vi "显示UI.vi"() -> ()   [LabVIEW 2016, in "国弘多参数.lvlib"]
uses:
  <vilib>/Utility/miscctls.llb/LVPointTypeDef.ctl
  <vilib>/Utility/config.llb/NI_LVConfig.lvlib
panel:
  out "运行状态":u16(ring) items=["空闲", "水样测试", "标样核查"]
  in  "叶绿素a校准":bool
  in  "停止":bool
  in  "标样核查":bool
  in  "水样测试":bool
  in  "open MB":bool
  in  "设置":bool
  in  "水温校准":bool
  in  "浊度校准":bool
  in  "溶解氧校准":bool
  in  "电导率校准":bool
  in  "pH校准":bool
  in  "探头校正返回":bool
  in  "探头校正":bool
  in  "浊度参数查询":bool
  in  "溶解氧参数查询":bool
  in  "电导率参数查询":bool
  in  "pH参数查询":bool
  out "检测值":T1
  in  "返回":bool
  in  "参数查询":bool
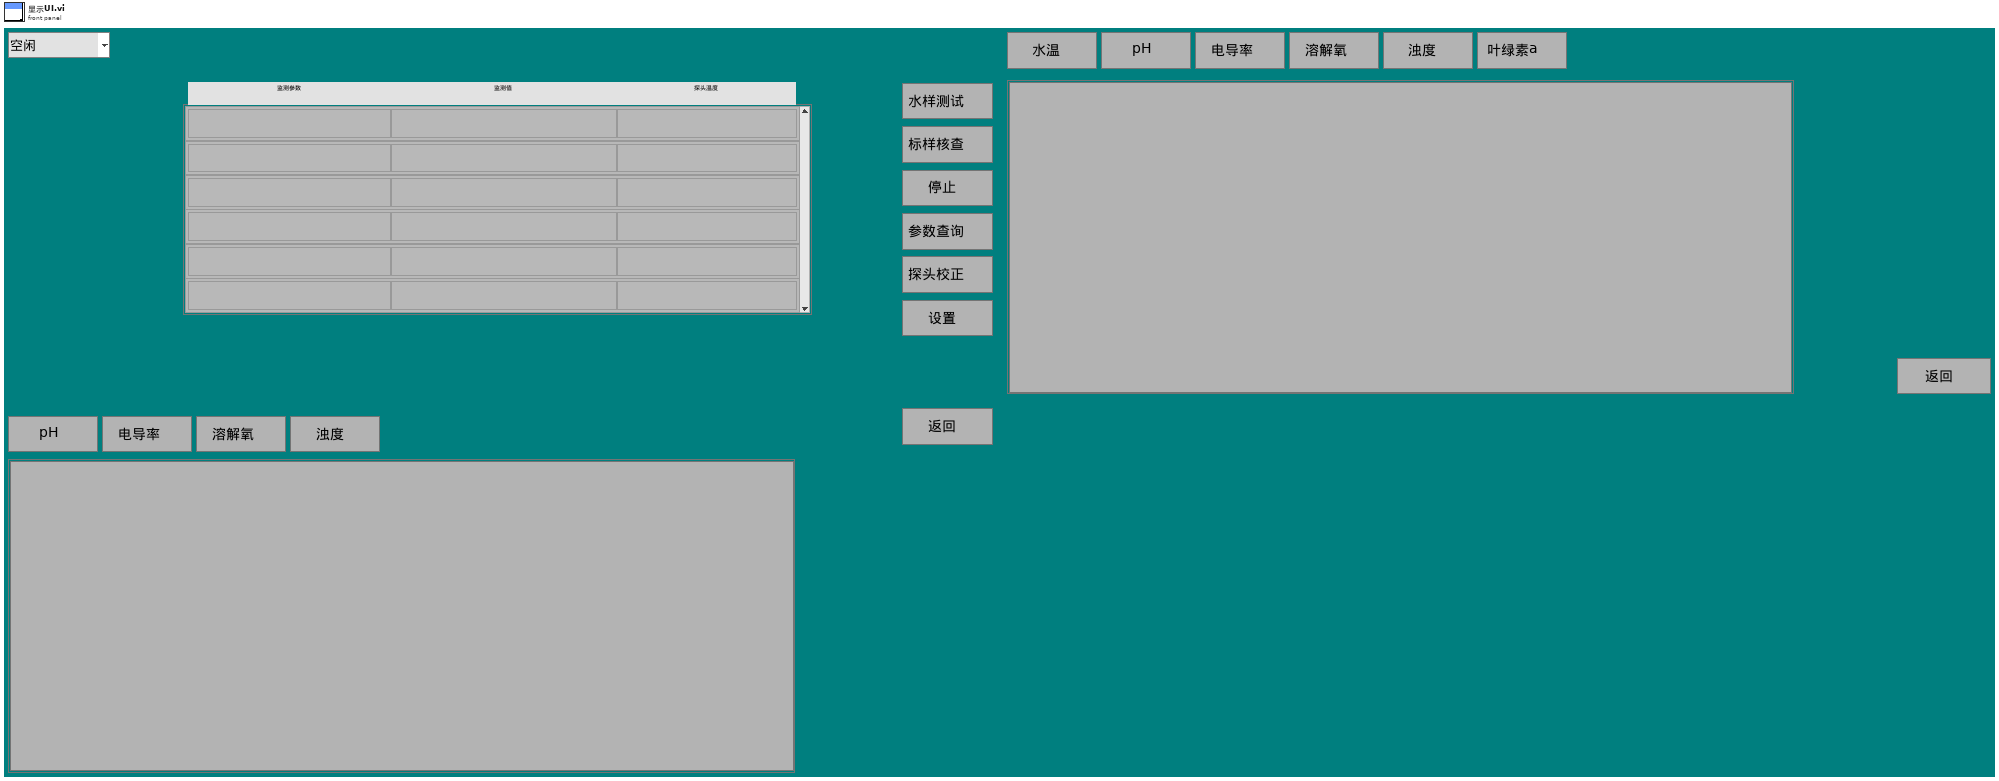
[diagram p1: front panel]
types:
  T1 = typedef "国弘多参数.lvlib/检测值.ctl" = cluster{"监测参数1":string, "浓度1":string, "探头温度1":string}[]
  T2 = typedef "LVPointTypeDef.ctl" = cluster{"Horizontal":i16, "Vertical":i16}
  T3 = cluster{"电极状态标志":u16, "电极型号标志":u16, "溶解氧测量值":sgl, "温度测量值":sgl, "溶解氧饱和度值":sgl, "盐度补偿值":sgl, "大气压补偿值":sgl, "溶解氧偏移修正值":sgl, "温度偏移修正值":sgl, "手动温度补偿值":sgl, "溶解氧电极零点":sgl, "溶解氧电极斜率":sgl, "第1点标准值记录":sgl, "第1点信号值记录":sgl, "第1点温度值记录":sgl, "第2点标准值记录":sgl, "第2点信号值记录":sgl, "第2点温度值记录":sgl, "命令滤波设定":u16, "温度模式":enum16{"ATC", "MTC"}, "生产批次":u16, "电极序号":u16, "串口地址":u16, "串口波特率":enum16{"9600", "19200", "115200"}, "串口校验位":enum16{"NONE", "ODD", "EVEN"}, "串口停止位":enum16{"1bit", "2bit"}, "第一点标准值":sgl, "第二点标准值":sgl}
  T4 = cluster{"电极状态标志":u16, "电极型号标志":u16, "酸碱度测量值":sgl, "温度测量值":sgl, "酸碱度信号值":sgl, "温度信号值":sgl, "酸碱度偏移修正值":sgl, "温度偏移修正值":sgl, "手动温度补偿值":sgl, "酸碱度电极零点":sgl, "酸碱度电极斜率":sgl, "第1点标准值记录":sgl, "第1点信号值记录":sgl, "第1点温度值记录":sgl, "第2点标准值记录":sgl, "第2点信号值记录":sgl, "第2点温度值记录":sgl, "命令滤波设定":u16, "温度模式":enum16{"ATC", "MTC"}, "生产批次":u16, "电极序号":u16, "串口地址":u16, "串口波特率":enum16{"9600", "19200", "115200"}, "串口校验位":enum16{"NONE", "ODD", "EVEN"}, "串口停止位":enum16{"1bit", "2bit"}, "第一点标准值":sgl, "第二点标准值":sgl}
  T5 = cluster{"电极状态标志":u16, "电极型号标志":u16, "浊度测量值":sgl, "温度测量值":sgl, "浊度信号值":sgl, "浊度偏移修正值":sgl, "温度偏移修正值":sgl, "手动温度补偿值":sgl, "浊度电极零点":sgl, "浊度电极斜率":sgl, "第1点标准值记录":sgl, "第1点信号值记录":sgl, "第1点温度值记录":sgl, "第2点标准值记录":sgl, "第2点信号值记录":sgl, "第2点温度值记录":sgl, "命令滤波设定":u16, "温度模式":enum16{"ATC", "MTC"}, "生产批次":u16, "电极序号":u16, "串口地址":u16, "串口波特率":enum16{"9600", "19200", "115200"}, "串口校验位":enum16{"NONE", "ODD", "EVEN"}, "串口停止位":enum16{"1bit", "2bit"}, "第一点标准值":sgl, "第二点标准值":sgl}
  T6 = cluster{"电极状态标志":u16, "电极型号标志":u16, "电导率测量值":sgl, "温度测量值":sgl, "电导率信号值":sgl, "温度信号值":sgl, "温度补偿系数":sgl, "电导率偏移修正值":sgl, "温度偏移修正值":sgl, "手动温度补偿值":sgl, "电导率电极零点":sgl, "电导率电极斜率":sgl, "命令滤波设定":u16, "温度模式":enum16{"ATC", "MTC"}, "生产批次":u16, "电极序号":u16, "串口地址":u16, "串口波特率":enum16{"9600", "19200", "115200"}, "串口校验位":enum16{"NONE", "ODD", "EVEN"}, "串口停止位":enum16{"1bit", "2bit"}, "第一点标准值":sgl, "第二点标准值":sgl}
  T7 = cluster{"监测参数1":string, "浓度1":string, "探头温度1":string}[]
  T8 = cluster{"CH":u16, "监测值":dbl, "监测信号值":dbl, "温度偏移修正值":sgl}
  T9 = typedef "NI_LVConfig.lvlib/Config Data RefNum.ctl" = refnum<k1>
  T10 = cluster{"baud rate (bps)":u32, "stop bits":u16, "parity":u16, "flow control":u16, "timeout":u32, "retries":i32}
  T11 = enum32{"Bad", "Idle", "Run top level", "Running"}
  T12 = cluster{"数据保存间隔":dbl, "水温标样值":dbl, "pH标样值":dbl, "溶解氧标样值":dbl, "电导率标样值":dbl, "浊度标样值":dbl}
  T13 = cluster{"Temp":bool, "pH":bool, "DO":bool, "Cond":bool, "Turb":bool, "叶绿素a启用":bool}
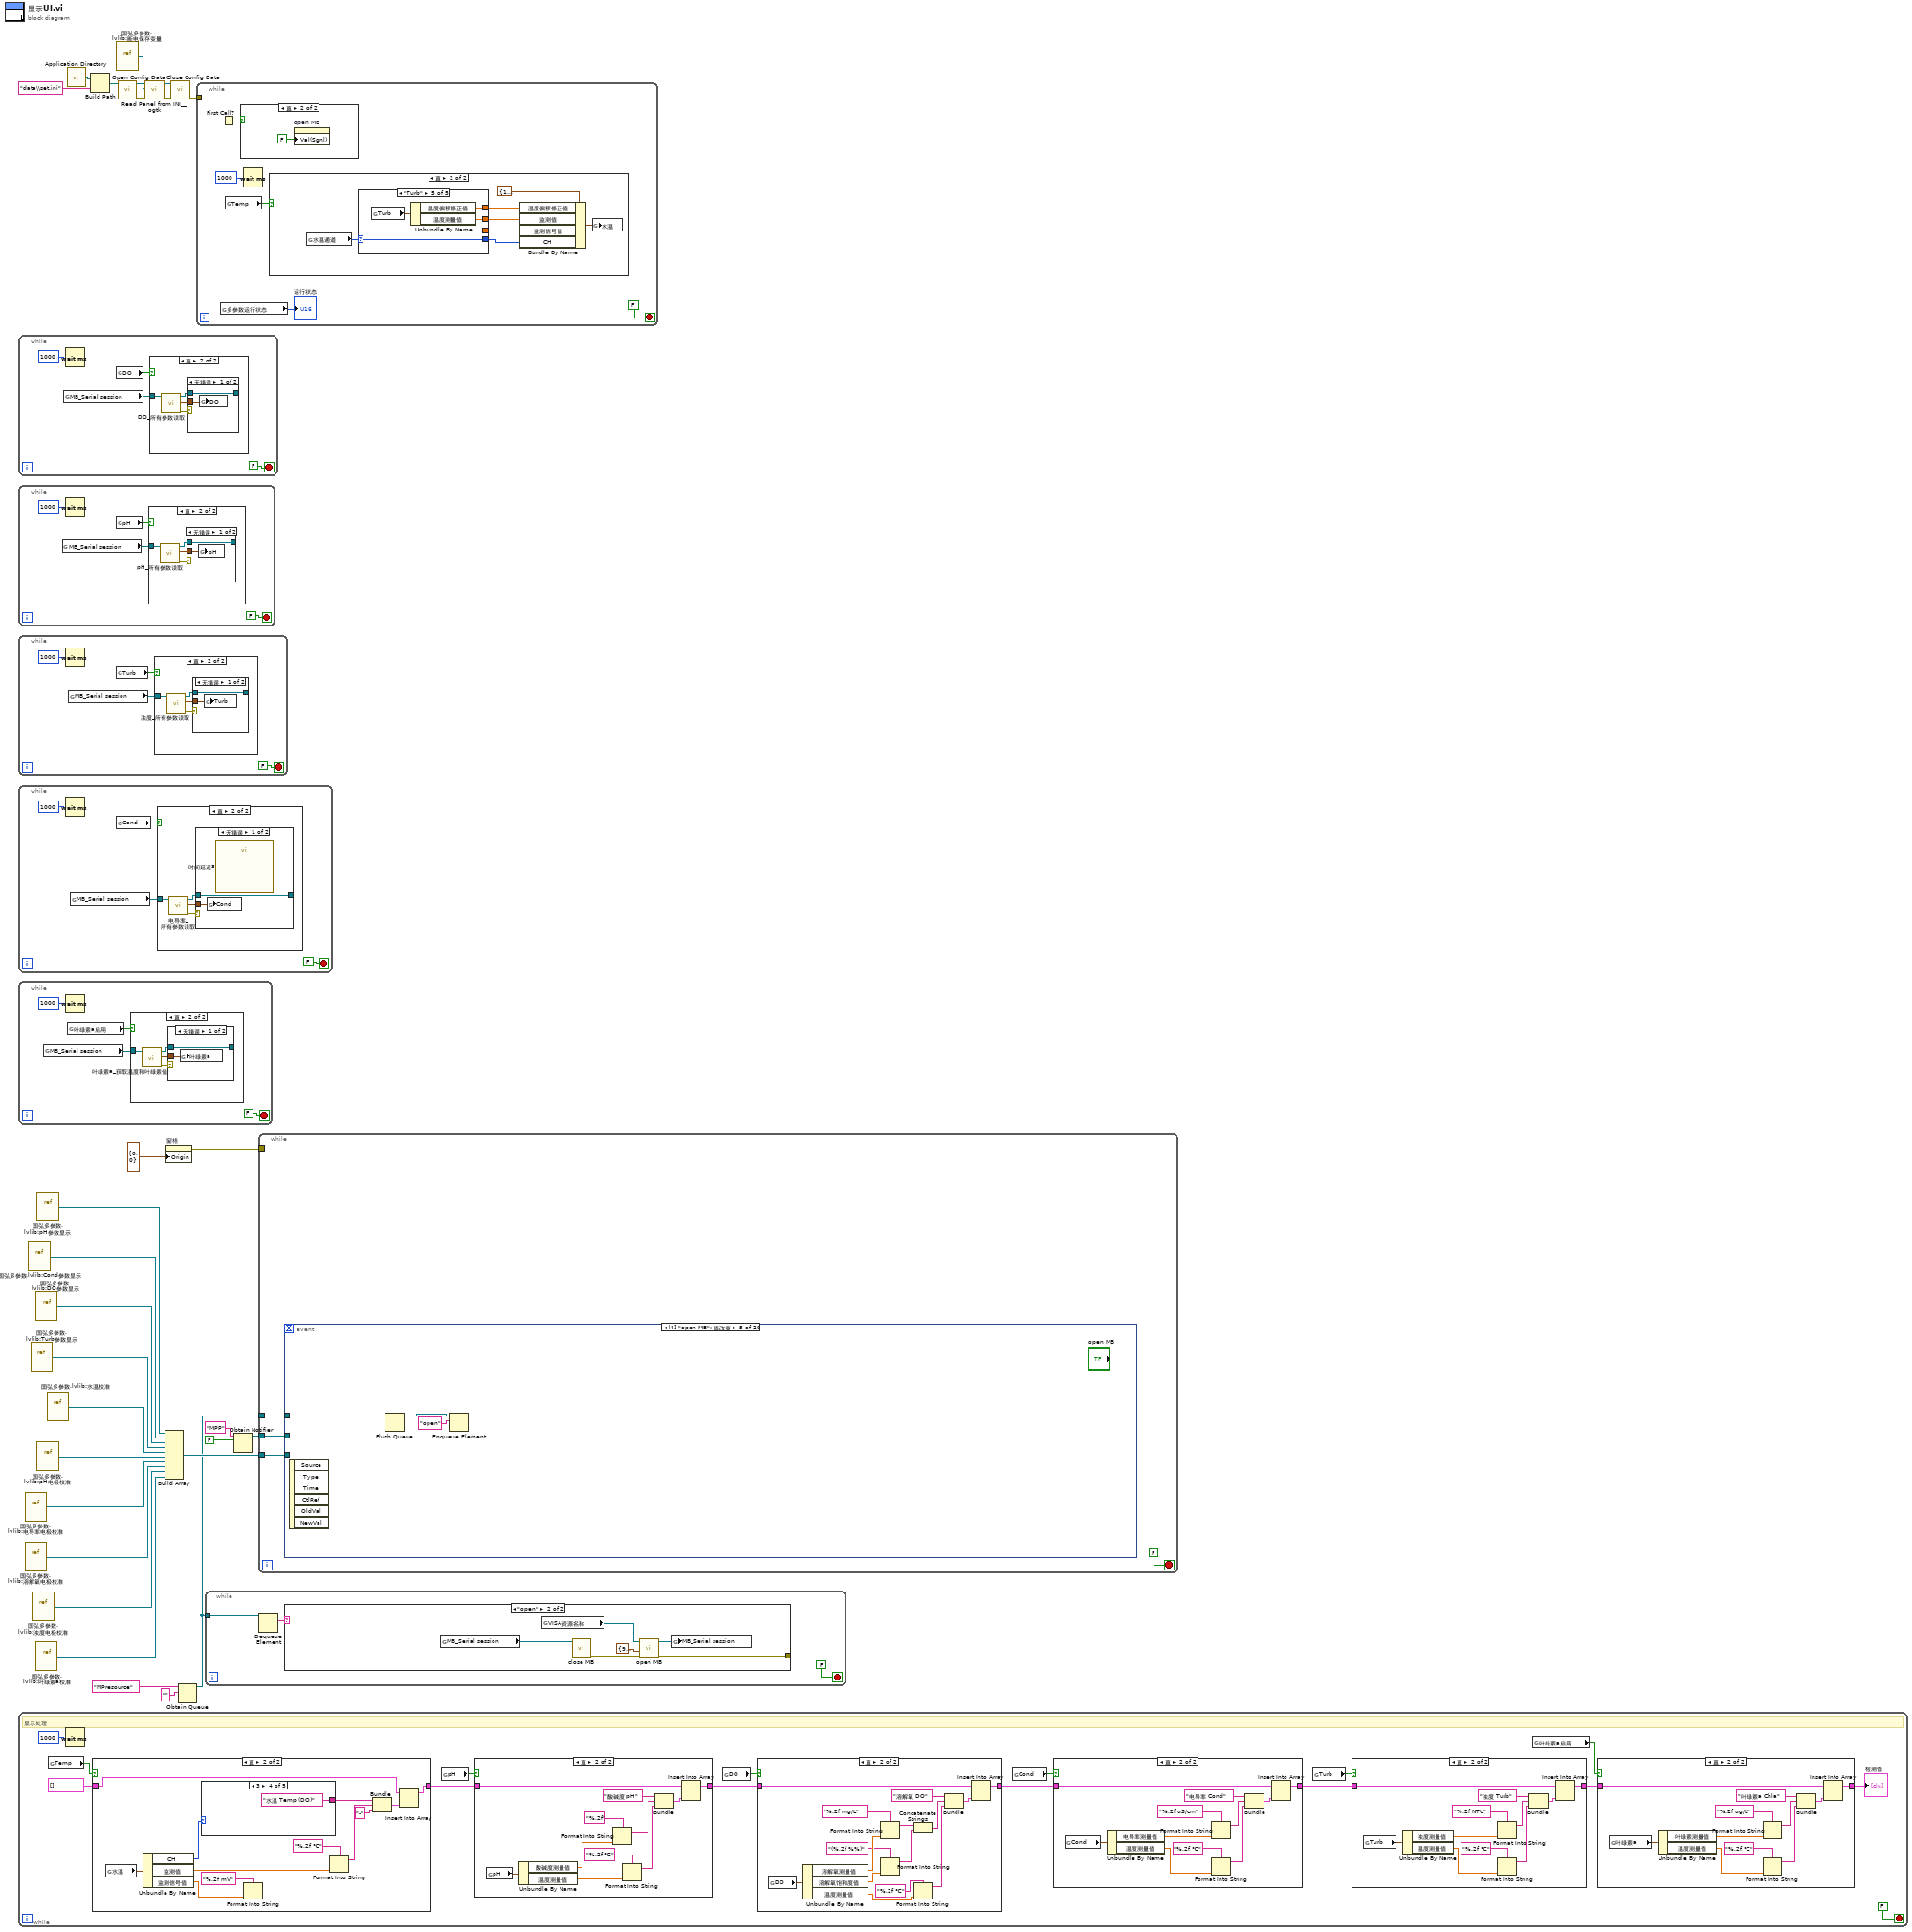
[diagram p0: block diagram]
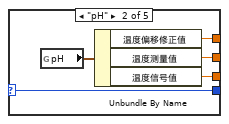
[diagram p15: hidden frame]
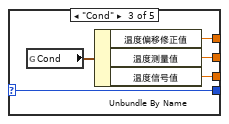
[diagram p16: hidden frame]
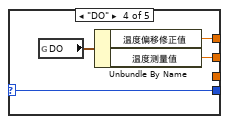
[diagram p17: hidden frame]
diagram:
  n1 = while {
    stop <- FALSE stop-if-true
    n2 = global read "过程全局变量.vi" "MB_Serial session"() -> (w29:refnum<class "MB_Master_Serial.lvclass">)
    n3 = Wait (ms)(milliseconds to wait=u32 1000 ("等待时间（毫秒）")) -> ()  [unwired: 1 out]
    n4 = global read "断电保存变量.vi" "DO"() -> (w30:bool)
    n5 = case shown="真" w30 {
      tunnel: w29 -> [_ w33]
      frame False {
      }
      frame True {
        n6 = call "DO_所有参数读取.vi"("MB_Serial session in"=w33) -> ("error out"=w35:errorcluster, "输出值"=w36:T3, "MB_Serial session out"=w34:refnum<class "MB_Master_Serial.lvclass">)  [unwired: 8 in]
        n7 = case shown="无错误" w35 {
          tunnel: w36 -> [w38 _]
          tunnel: w34 -> [w37 w39]
          tunnel: [w37 w39] -> _
          frame No Error {
            n8 = global write "过程全局变量.vi" "DO"(w38) -> ()
          }
          frame Error {
          }
        }
      }
    }
  }
  n9 = while {
    stop <- FALSE stop-if-true
    n10 = global read "过程全局变量.vi" "MB_Serial session"() -> (w41:refnum<class "MB_Master_Serial.lvclass">)
    n11 = Wait (ms)(milliseconds to wait=u32 1000 ("等待时间（毫秒）")) -> ()  [unwired: 1 out]
    n12 = global read "断电保存变量.vi" "pH"() -> (w42:bool)
    n13 = case shown="真" w42 {
      tunnel: w41 -> [_ w44]
      frame False {
      }
      frame True {
        n14 = call "pH_所有参数读取.vi"("MB_Serial session in"=w44) -> ("error out"=w46:errorcluster, "输出值"=w47:T4, "MB_Serial session out"=w45:refnum<class "MB_Master_Serial.lvclass">)  [unwired: 8 in]
        n15 = case shown="无错误" w46 {
          tunnel: w47 -> [w49 _]
          tunnel: w45 -> [w48 w50]
          tunnel: [w48 w50] -> _
          frame No Error {
            n16 = global write "过程全局变量.vi" "pH"(w49) -> ()
          }
          frame Error {
          }
        }
      }
    }
  }
  n17 = while {
    stop <- FALSE stop-if-true
    n18 = Wait (ms)(milliseconds to wait=u32 1000 ("等待时间（毫秒）")) -> ()  [unwired: 1 out]
    n19 = global read "过程全局变量.vi" "MB_Serial session"() -> (w52:refnum<class "MB_Master_Serial.lvclass">)
    n20 = global read "断电保存变量.vi" "Turb"() -> (w53:bool)
    n21 = case shown="真" w53 {
      tunnel: w52 -> [_ w55]
      frame False {
      }
      frame True {
        n22 = call "浊度_所有参数读取.vi"("MB_Serial session in"=w55) -> ("error out"=w57:errorcluster, "输出值"=w58:T5, "MB_Serial session out"=w56:refnum<class "MB_Master_Serial.lvclass">)  [unwired: 8 in]
        n23 = case shown="无错误" w57 {
          tunnel: w58 -> [w60 _]
          tunnel: w56 -> [w59 w61]
          tunnel: [w59 w61] -> _
          frame No Error {
            n24 = global write "过程全局变量.vi" "Turb"(w60) -> ()
          }
          frame Error {
          }
        }
      }
    }
  }
  n25 = while {
    stop <- FALSE stop-if-true
    n26 = Wait (ms)(milliseconds to wait=u32 1000 ("等待时间（毫秒）")) -> ()  [unwired: 1 out]
    n27 = global read "过程全局变量.vi" "MB_Serial session"() -> (w63:refnum<class "MB_Master_Serial.lvclass">)
    n28 = global read "断电保存变量.vi" "Cond"() -> (w64:bool)
    n29 = case shown="真" w64 {
      tunnel: w63 -> [_ w66]
      frame False {
      }
      frame True {
        n30 = call "电导率_所有参数读取.vi"("MB_Serial session in"=w66) -> ("error out"=w68:errorcluster, "输出值"=w69:T6, "MB_Serial session out"=w67:refnum<class "MB_Master_Serial.lvclass">)  [unwired: 8 in]
        n31 = case shown="无错误" w68 {
          tunnel: w69 -> [w71 _]
          tunnel: [w70 w72] -> _
          tunnel: w67 -> [w70 w72]
          frame No Error {
            n32 = global write "过程全局变量.vi" "Cond"(w71) -> ()
            n33 = call "时间延迟3"() -> ()  [unwired: 11 in, 1 out]
          }
          frame Error {
          }
        }
      }
    }
  }
  n34 = while {
    stop <- FALSE stop-if-true
    n35 = global read "过程全局变量.vi" "MB_Serial session"() -> (w75:refnum<class "MB_Master_Serial.lvclass">)
    n36 = Wait (ms)(milliseconds to wait=u32 1000 ("等待时间（毫秒）")) -> ()  [unwired: 1 out]
    n37 = global read "断电保存变量.vi" "叶绿素a启用"() -> (w74:bool)
    n38 = case shown="真" w74 {
      tunnel: w75 -> [_ w77]
      frame False {
      }
      frame True {
        n39 = call "叶绿素a_获取温度和叶绿素值.vi"("MB_Serial session in"=w77) -> ("error out"=w79:errorcluster, "输出值"=w80:cluster{"温度测量值":sgl, "叶绿素测量值":sgl, "错误标志":u16}, "MB_Serial session out"=w78:refnum<class "MB_Master_Serial.lvclass">)  [unwired: 8 in]
        n40 = case shown="无错误" w79 {
          tunnel: w80 -> [w82 _]
          tunnel: w78 -> [w81 w83]
          tunnel: [w81 w83] -> _
          frame No Error {
            n41 = global write "过程全局变量.vi" "叶绿素a"(w82) -> ()
          }
          frame Error {
          }
        }
      }
    }
  }
  n42 = while {
    stop <- FALSE stop-if-true
    # "显示处理"
    n43 = global read "断电保存变量.vi" "Temp"() -> (w96:bool)
    n44 = Wait (ms)(milliseconds to wait=u32 1000 ("等待时间（毫秒）")) -> ()  [unwired: 1 out]
    n45 = case shown="真" w96 {
      tunnel: [w163 w164] -> w93
      tunnel: T7 [] ("数组") -> [w163 w165]
      frame False {
      }
      frame True {
        n46 = global read "过程全局变量.vi" "水温"() -> (w175:T8)
        n47 = Unbundle By Name(w175) -> ("CH"=w170:u16, "监测值"=w173:dbl, "监测信号值"=w171:dbl)
        n48 = case shown="3" w170 {
          tunnel: ["水温 Temp" ("监测参数1") "水温 Temp (pH)" ("监测参数1") "水温 Temp (Cond)" ("监测参数1") "水温 Temp (DO)" ("监测参数1") "水温 Temp (Turb)" ("监测参数1")] -> w169
          frame 0, Default {
          }
          frame 1 {
          }
          frame 2 {
          }
          frame 3 {
          }
          frame 4 {
          }
        }
        n49 = Format Into String(format string="%.2f mV" ("格式字符串"), w171) -> ()  [unwired: 2 in, 2 out]
        n50 = Format Into String(format string="%.2f ℃" ("格式字符串"), w173) -> (resulting string=w168:string)  [unwired: 2 in, 1 out]
        n51 = Bundle("监测参数1"=w169, w168, "探头温度1"="-") -> (w166:cluster{"监测参数1":string, string, "探头温度1":string})  [unwired: 1 in]
        n52 = Insert Into Array(array=w165, new element=w166) -> (w164:T7)  [unwired: 1 in]
      }
    }
    n53 = global read "断电保存变量.vi" "pH"() -> (w94:bool)
    n54 = case shown="真" w94 {
      tunnel: [w151 w152] -> w91
      tunnel: w93 -> [w151 w154]
      frame False {
      }
      frame True {
        n55 = global read "过程全局变量.vi" "pH"() -> (w162:T4)
        n56 = Unbundle By Name(w162) -> ("酸碱度测量值"=w161:sgl, "温度测量值"=w159:sgl)
        n57 = Format Into String(format string="%.2f" ("格式字符串"), w161) -> (resulting string=w155:string)  [unwired: 2 in, 1 out]
        n58 = Format Into String(format string="%.2f ℃" ("格式字符串"), w159) -> (resulting string=w157:string)  [unwired: 2 in, 1 out]
        n59 = Bundle("监测参数2"="酸碱度 pH", w155, w157) -> (w153:cluster{"监测参数2":string, string, string})  [unwired: 1 in]
        n60 = Insert Into Array(array=w154, new element=w153) -> (w152:T7)  [unwired: 1 in]
      }
    }
    n61 = global read "断电保存变量.vi" "DO"() -> (w92:bool)
    n62 = case shown="真" w92 {
      tunnel: [w135 w136] -> w88
      tunnel: w91 -> [w135 w137]
      frame False {
      }
      frame True {
        n63 = global read "过程全局变量.vi" "DO"() -> (w146:T3)
        n64 = Unbundle By Name(w146) -> ("溶解氧测量值"=w147:sgl, "溶解氧饱和度值"=w144:sgl, "温度测量值"=w149:sgl)
        n65 = Format Into String(format string="%.2f mg/L" ("格式字符串"), w147) -> (resulting string=w143:string)  [unwired: 2 in, 1 out]
        n66 = Format Into String(format string="(%.2f %%)" ("格式字符串"), w144) -> (resulting string=w142:string)  [unwired: 2 in, 1 out]
        n67 = Concatenate Strings(w143, w142) -> (w141:string)
        n68 = Format Into String(format string="%.2f ℃" ("格式字符串"), w149) -> (resulting string=w139:string)  [unwired: 2 in, 1 out]
        n69 = Bundle("监测参数2"="溶解氧 DO", w141, w139) -> (w138:cluster{"监测参数2":string, string, string})  [unwired: 1 in]
        n70 = Insert Into Array(array=w137, new element=w138) -> (w136:T7)  [unwired: 1 in]
      }
    }
    n71 = global read "断电保存变量.vi" "Cond"() -> (w90:bool)
    n72 = case shown="真" w90 {
      tunnel: w88 -> [w123 w126]
      tunnel: [w123 w124] -> w87
      frame False {
      }
      frame True {
        n73 = global read "过程全局变量.vi" "Cond"() -> (w134:T6)
        n74 = Unbundle By Name(w134) -> ("电导率测量值"=w133:sgl, "温度测量值"=w131:sgl)
        n75 = Format Into String(format string="%.2f uS/cm" ("格式字符串"), w133) -> (resulting string=w127:string)  [unwired: 2 in, 1 out]
        n76 = Format Into String(format string="%.2f ℃" ("格式字符串"), w131) -> (resulting string=w128:string)  [unwired: 2 in, 1 out]
        n77 = Bundle("监测参数2"="电导率 Cond", w127, w128) -> (w125:cluster{"监测参数2":string, string, string})  [unwired: 1 in]
        n78 = Insert Into Array(array=w126, new element=w125) -> (w124:T7)  [unwired: 1 in]
      }
    }
    n79 = global read "断电保存变量.vi" "Turb"() -> (w89:bool)
    n80 = case shown="真" w89 {
      tunnel: w87 -> [w111 w114]
      tunnel: [w111 w112] -> w86
      frame False {
      }
      frame True {
        n81 = global read "过程全局变量.vi" "Turb"() -> (w118:T5)
        n82 = Unbundle By Name(w118) -> ("浊度测量值"=w119:sgl, "温度测量值"=w121:sgl)
        n83 = Format Into String(format string="%.2f NTU" ("格式字符串"), w119) -> (resulting string=w116:string)  [unwired: 2 in, 1 out]
        n84 = Format Into String(format string="%.2f ℃" ("格式字符串"), w121) -> (resulting string=w117:string)  [unwired: 2 in, 1 out]
        n85 = Bundle("监测参数2"="浊度 Turb", w116, w117) -> (w113:cluster{"监测参数2":string, string, string})  [unwired: 1 in]
        n86 = Insert Into Array(array=w114, new element=w113) -> (w112:T7)  [unwired: 1 in]
      }
    }
    n87 = global read "断电保存变量.vi" "叶绿素a启用"() -> (w84:bool)
    n88 = case shown="真" w84 {
      tunnel: w86 -> [w99 w102]
      tunnel: [w99 w100] -> w85
      frame False {
      }
      frame True {
        n89 = global read "过程全局变量.vi" "叶绿素a"() -> (w106:cluster{"温度测量值":sgl, "叶绿素测量值":sgl, "错误标志":u16})
        n90 = Unbundle By Name(w106) -> ("叶绿素测量值"=w107:sgl, "温度测量值"=w109:sgl)
        n91 = Format Into String(format string="%.2f ug/L" ("格式字符串"), w107) -> (resulting string=w104:string)  [unwired: 2 in, 1 out]
        n92 = Format Into String(format string="%.2f ℃" ("格式字符串"), w109) -> (resulting string=w105:string)  [unwired: 2 in, 1 out]
        n93 = Bundle("监测参数2"="叶绿素a Chla", w104, w105) -> (w101:cluster{"监测参数2":string, string, string})  [unwired: 1 in]
        n94 = Insert Into Array(array=w102, new element=w101) -> (w100:T7)  [unwired: 1 in]
      }
    }
    "检测值" <- w85
  }
  n95 = vi-ref "国弘多参数.lvlib:电导率电极校准.vi"() -> (w19:refnum<vi>)
  n96 = vi-ref "国弘多参数.lvlib:溶解氧电极校准.vi"() -> (w18:refnum<vi>)
  n97 = vi-ref "国弘多参数.lvlib:Cond参数显示.vi"() -> (w25:refnum<vi>)
  n98 = vi-ref "国弘多参数.lvlib:Turb参数显示.vi"() -> (w23:refnum<vi>)
  n99 = vi-ref "国弘多参数.lvlib:浊度电极校准.vi"() -> (w17:refnum<vi>)
  n100 = vi-ref "国弘多参数.lvlib:DO参数显示.vi"() -> (w24:refnum<vi>)
  n101 = vi-ref "国弘多参数.lvlib:叶绿素a校准.vi"() -> (w7:refnum<vi>)
  n102 = vi-ref "国弘多参数.lvlib:pH参数显示.vi"() -> (w26:refnum<vi>)
  n103 = vi-ref "国弘多参数.lvlib:pH电极校准.vi"() -> (w20:refnum<vi>)
  n104 = vi-ref "国弘多参数.lvlib:水温校准.vi"() -> (w21:refnum<vi>)
  n105 = call <vilib>:"Application Directory.vi"() -> ("Application Directory"=w12:path)
  n106 = Build Path(base path=w12, name or relative path="data\\set.ini" ("名称或相对路径")) -> (appended path=w11:path)
  n107 = vi-ref "国弘多参数.lvlib:断电保存变量.vi"() -> (w9:refnum<vi>)
  n108 = call <vilib>:"Open Config Data.vi"("configuration file path"=w11) -> ("error out"=w15:errorcluster, "refnum"=w16:T9)  [unwired: 8 in, 1 out]
  n109 = call <userlib>:"Read Panel from INI__ogtk.vi"("error in (no error)"=w15, "VI ref"=w9, "refnum"=w16) -> ("error out"=w13:errorcluster, "refnum out"=w14:T9)  [unwired: 7 in]
  n110 = Build Array(w26, w25, w24, w23, w21, w20, w19, w18, w17, w7) -> (w22:refnum<vi>[])
  n111 = property on="窗格" class="Pane"("Origin"=T2 {"Horizontal"=0, "Vertical"=0} ("原点")) -> (error out=w28:errorcluster)  [unwired: 2 in, 1 out]
  n112 = call <vilib>:"Close Config Data.vi"("error in (no error)"=w13, "refnum"=w14) -> ("error out"=w8:errorcluster)  [unwired: 8 in, 1 out]
  n113 = Obtain Queue(name (unnamed)="MPresource" ("名称（未命名）"), element data type="" ("名称（未命名）")) -> (queue out=w1:refnum<queue>)  [unwired: 3 in, 2 out]
  n114 = while {
    tunnel: w8 -> [_]
    stop <- FALSE stop-if-true
    n115 = First Call?() -> (First Call?: T/F=w183:bool)
    n116 = global read "过程全局变量.vi" "多参数运行状态"() -> (→"运行状态":u16)
    n117 = global read "断电保存变量.vi" "Temp"() -> (w182:bool)
    n118 = case shown="真" w183 {
      frame False {
      }
      frame True {
        n119 = property on="open MB" class="Bool (严格)"("Val(Sgnl)"=FALSE ("值(信号)")) -> ()  [unwired: 2 in, 2 out]
      }
    }
    n120 = Wait (ms)(milliseconds to wait=u32 1000 ("等待时间（毫秒）")) -> ()  [unwired: 1 out]
    n121 = case shown="真" w182 {
      frame False {
      }
      frame True {
        n122 = global read "断电保存变量.vi" "水温通道"() -> (w192:enum16{"NULL", "pH", "Cond", "DO", "Turb"})
        n123 = case shown="\"Turb\"" w192 {
          selector: w192 -> [w193 w198 w203 w207 w211]
          tunnel: [w193 w198 w203 w207 w211] -> w191
          tunnel: [_ w196 w201 w205 w209] -> w190
          tunnel: [_ w195 w200 _ _] -> w189
          tunnel: [_ w194 w199 w204 w208] -> w186
          frame "NULL", Default {
          }
          frame "pH" {
            n124 = global read "过程全局变量.vi" "pH"() -> (w197:T4)
            n125 = Unbundle By Name(w197) -> ("温度偏移修正值"=w194:sgl, "温度测量值"=w196:sgl, "温度信号值"=w195:sgl)
          }
          frame "Cond" {
            n126 = global read "过程全局变量.vi" "Cond"() -> (w202:T6)
            n127 = Unbundle By Name(w202) -> ("温度偏移修正值"=w199:sgl, "温度测量值"=w201:sgl, "温度信号值"=w200:sgl)
          }
          frame "DO" {
            n128 = global read "过程全局变量.vi" "DO"() -> (w206:T3)
            n129 = Unbundle By Name(w206) -> ("温度偏移修正值"=w204:sgl, "温度测量值"=w205:sgl)
          }
          frame "Turb" {
            n130 = global read "过程全局变量.vi" "Turb"() -> (w210:T5)
            n131 = Unbundle By Name(w210) -> ("温度偏移修正值"=w208:sgl, "温度测量值"=w209:sgl)
          }
        }
        n132 = Bundle By Name(cluster=T8 {"CH"=1, "监测值"=0.0, "监测信号值"=0.0, "温度偏移修正值"=0.0} ("水温"), "温度偏移修正值"=w186, "监测值"=w190, "监测信号值"=w189, "CH"=w191) -> (w188:T8)
        n133 = global write "过程全局变量.vi" "水温"(w188) -> ()
      }
    }
  }
  n134 = while {
    tunnel: w1 -> [w214]
    stop <- FALSE stop-if-true
    n135 = Dequeue Element(queue=w214) -> (element=w213:string)  [unwired: 2 in, 3 out]
    n136 = case shown="\"open\"" w213 {
      tunnel: [_ w216] -> _
      frame "假", Default {
      }
      frame "open" {
        n137 = global read "过程全局变量.vi" "MB_Serial session"() -> (w221:refnum<class "MB_Master_Serial.lvclass">)
        n138 = global read "断电保存变量.vi" "VISA资源名称"() -> (w218:refnum<visa-resource-name>)
        n139 = call "close MB.vi"("MB_Serial session"=w221) -> ("error out"=w220:errorcluster)  [unwired: 10 in]
        n140 = call "open MB.vi"("error in (no error)"=w220, "Serial Config"=T10 {"baud rate (bps)"=9600, "stop bits"=10, "parity"=0, "flow control"=0, "timeout"=1000, "retries"=1}, "VISA资源名称"=w218) -> ("error out"=w216:errorcluster, "MB_Serial session"=w219:refnum<class "MB_Master_Serial.lvclass">)  [unwired: 7 in]
        n141 = global write "过程全局变量.vi" "MB_Serial session"(w219) -> ()
      }
    }
  }
  n142 = Obtain Notifier(name (unnamed)="MPP" ("名称（未命名）"), notification data type=FALSE) -> (notifier out=w4:refnum<notifier>)  [unwired: 2 in, 2 out]
  n143 = while {
    tunnel: w28 -> [_]
    tunnel: w22 -> [w224]
    tunnel: w4 -> [w223]
    tunnel: w1 -> [w222]
    stop <- FALSE stop-if-true
    n144 = event shown="[4] \"open MB\": 值改变" {
      selector: _ -> [_ _ _ _ _ _ _ _ _ _ _ _ _ _ _ _ _ _ _ _]
      dyn-events: _ -> [_ _ _ _ _ _ _ _ _ _ _ _ _ _ _ _ _ _ _ _]
      timeout: _ -> [_ _ _ _ _ _ _ _ _ _ _ _ _ _ _ _ _ _ _ _]
      tunnel: w224 -> [_ _ _ _ _ _ w284 w297 w309 w317 w329 w341 w353 w365 w377 w389 w401 w413 w425 w437]
      tunnel: w223 -> [_ _ _ w257 _ _ _ _ _ _ _ _ _ _ _ _ _ _ _ _]
      tunnel: w222 -> [_ _ _ _ w260 _ _ _ _ _ _ _ _ _ _ _ _ _ _ _]
      event Timeout {
        n145 = event-data() -> ()  [unwired: 1 in, 3 out]
      }
      event "水样测试": Value Change {
        n146 = event-data() -> ()  [unwired: 1 in, 6 out]
        n147 = call "水样测试配置.vi"() -> ("确认输出"=w227:bool, "水样测定时间输出"=w226:dbl)  [unwired: 10 in]
        n148 = case shown="真" w227 {
          tunnel: w226 -> [_ w230]
          frame False {
          }
          frame True {
            n149 = vi-ref "国弘多参数.lvlib:水样测试.vi"() -> (w231:refnum<vi>)
            n150 = property class="VI"(reference=w231) -> ("Name"=w235:string, "Exec.State"=w233:T11)  [unwired: 1 in, 2 out]
            n151 = Open VI Reference(type specifier VI Refnum (for type only)=refnum<vi> refnum, vi path=w235, options=128 ("选项")) -> (vi reference=w236:refnum<vi>)  [unwired: 3 in, 1 out]
            n152 = case shown="\"Idle\"" w233 {
              tunnel: [w237 w241] -> w232
              tunnel: w236 -> [w237 w240]
              tunnel: w230 -> [_ w239]
              tunnel: "hd" ("数据标记表") -> [_ w238]
              frame "Bad", Default {
              }
              frame "Idle" {
                n153 = call-by-ref "开始异步调用"(reference=w240, "数据标记表"=w238, "水样测试时间"=w239) -> (reference out=w241:refnum<vi>)  [unwired: 11 in, 1 out]
              }
            }
            n154 = Close Reference(reference=w232) -> ()  [unwired: 1 in, 1 out]
          }
        }
      }
      event "标样核查": Value Change {
        n155 = event-data() -> ()  [unwired: 1 in, 6 out]
        n156 = call "标样核查配置.vi"() -> ("确认输出"=w243:bool, "标样核查配置"=w242:T12)  [unwired: 10 in]
        n157 = case shown="真" w243 {
          tunnel: w242 -> [_ w244]
          frame False {
          }
          frame True {
            n158 = vi-ref "国弘多参数.lvlib:标样核查.vi"() -> (w245:refnum<vi>)
            n159 = property class="VI"(reference=w245) -> ("Name"=w250:string, "Exec.State"=w247:T11)  [unwired: 1 in, 2 out]
            n160 = Open VI Reference(type specifier VI Refnum (for type only)=refnum<vi> refnum, vi path=w250, options=128 ("选项")) -> (vi reference=w251:refnum<vi>)  [unwired: 3 in, 1 out]
            n161 = case shown="\"Idle\"" w247 {
              tunnel: [w252 w255] -> w246
              tunnel: w251 -> [w252 w254]
              tunnel: w244 -> [_ w253]
              frame "Bad", Default {
              }
              frame "Idle" {
                n162 = call-by-ref "开始异步调用"(reference=w254, "标样核查配置"=w253) -> (reference out=w255:refnum<vi>)  [unwired: 12 in, 1 out]
              }
            }
            n163 = Close Reference(reference=w246) -> ()  [unwired: 1 in, 1 out]
          }
        }
      }
      event "停止": Value Change {
        n164 = event-data() -> ()  [unwired: 1 in, 6 out]
        n165 = Send Notification(notification=TRUE ("通知"), notifier=w257) -> ()  [unwired: 1 in, 2 out]
      }
      event "open MB": Value Change {
        n166 = event-data() -> ()  [unwired: 1 in, 6 out]
        n167 = Flush Queue(queue=w260) -> (queue out=w259:refnum<queue>)  [unwired: 1 in, 2 out]
        n168 = Enqueue Element(queue=w259, element="open" ("元素")) -> ()  [unwired: 2 in, 3 out]
      }
      event "设置": Value Change {
        n169 = event-data() -> ()  [unwired: 1 in, 6 out]
        n170 = flat-sequence {
          frame #0 {
            n171 = call "配置.vi"() -> ("启用参数"=w267:T13, "串口输出"=w268:refnum<visa-resource-name>)  [unwired: 10 in]
            n172 = global write "断电保存变量.vi" "VISA资源名称"(w268) -> ()
            n173 = Unbundle By Name(w267) -> ("Temp"=w262:bool, "pH"=w263:bool, "DO"=w264:bool, "Cond"=w265:bool, "Turb"=w266:bool, "叶绿素a启用"=w261:bool)
            n174 = global write "断电保存变量.vi" "pH"(w263) -> ()
            n175 = global write "断电保存变量.vi" "DO"(w264) -> ()
            n176 = global write "断电保存变量.vi" "Cond"(w265) -> ()
            n177 = global write "断电保存变量.vi" "Turb"(w266) -> ()
            n178 = global write "断电保存变量.vi" "Temp"(w262) -> ()
            n179 = global write "断电保存变量.vi" "叶绿素a启用"(w261) -> ()
          }
          frame #1 {
            n180 = call <vilib>:"Application Directory.vi"() -> ("Application Directory"=w278:path)
            n181 = Build Path(base path=w278, name or relative path="data\\set.ini" ("名称或相对路径")) -> (appended path=w277:path)
            n182 = call <vilib>:"Open Config Data.vi"("configuration file path"=w277) -> ("error out"=w281:errorcluster, "refnum"=w282:T9)  [unwired: 8 in, 1 out]
            n183 = vi-ref "国弘多参数.lvlib:断电保存变量.vi"() -> (w275:refnum<vi>)
            n184 = call <userlib>:"Write Panel to INI__ogtk.vi"("error in (no error)"=w281, "VI ref"=w275, "refnum"=w282) -> ("error out"=w279:errorcluster, "refnum out"=w280:T9)  [unwired: 7 in]
            n185 = call <vilib>:"Close Config Data.vi"("error in (no error)"=w279, "refnum"=w280) -> ("error out"=w271:errorcluster, "file path"=w272:path)  [unwired: 8 in]
            n186 = Open/Create/Replace File(file path (use dialog)=w272, error in=w271) -> (refnum out=w273:refnum<file>, error out=w274:errorcluster)  [unwired: 4 in, 1 out]
            n187 = Flush File(refnum=w273, error in=w274) -> (refnum out=w269:refnum<file>, error out=w270:errorcluster)
            n188 = Close File(refnum=w269, error in=w270) -> ()  [unwired: 2 out]
          }
          frame #2 {
            n189 = property on="open MB" class="Bool (严格)"("Val(Sgnl)"=FALSE ("值(信号)")) -> ()  [unwired: 2 in, 2 out]
          }
        }
      }
      event "探头校正返回": Value Change {
        n190 = event-data() -> ()  [unwired: 1 in, 6 out]
        n191 = property on="窗格" class="Pane"("Origin"=T2 {"Horizontal"=0, "Vertical"=0} ("原点")) -> ()  [unwired: 2 in, 2 out]
        n192 = disable-structure shown="禁用" {
          disable-tunnel: w284 -> [w286 _]
          frame Disabled {
            n193 = for {
              tunnel: w286 -> [w289] mode=indexing
              n194 = property class="VI"(reference=w289) -> (reference out=w287:refnum<vi>, "Exec.State"=w288:T11)  [unwired: 1 in, 1 out]
              n195 = case shown="\"Run top level\"" w288 {
                tunnel: w287 -> [_ _ w290 w291]
                frame "Bad", Default {
                }
                frame "Idle" {
                }
                frame "Run top level" {
                  n196 = invoke class="VI" method="Abort VI"(reference=w290) -> ()  [unwired: 2 in, 3 out]
                }
                frame "Running" {
                  n197 = invoke class="VI" method="Abort VI"(reference=w291) -> ()  [unwired: 2 in, 3 out]
                }
              }
            }
          }
          frame Enabled {
          }
        }
      }
      event "探头校正": Value Change {
        n198 = event-data() -> ()  [unwired: 1 in, 6 out]
        n199 = property on="窗格" class="Pane"("Origin"=T2 {"Horizontal"=1656, "Vertical"=0} ("原点")) -> ()  [unwired: 2 in, 2 out]
        n200 = Index Array(array=w297, index=4 ("索引")) -> (element=w298:refnum<vi>)
        n201 = property class="VI"(reference=w298) -> (reference out=w293:refnum<vi>, "Exec.State"=w292:T11)  [unwired: 1 in, 1 out]
        n202 = case shown="\"Bad\", 默认" w292 {
          tunnel: [w300 w302] -> w296
          tunnel: w293 -> [w300 w301]
          frame "Bad", Default {
          }
          frame "Idle" {
            n203 = invoke class="VI" method="Run VI"(reference=w301, "Wait until done"=FALSE ("结束前等待"), "Auto Dispose Ref"=FALSE ("自动销毁引用")) -> (reference out=w302:refnum<vi>)  [unwired: 2 in, 4 out]
          }
        }
        n204 = invoke on="探头校准子面板" class="SubPnl" method="Remove VI"() -> (error out=w295:errorcluster)  [unwired: 3 in, 2 out]
        n205 = invoke on="探头校准子面板" class="SubPnl" method="Insert VI"(error in=w295, "VI Ref"=w296) -> ()  [unwired: 2 in, 4 out]
      }
      event "参数查询": Value Change {
        n206 = event-data() -> ()  [unwired: 1 in, 6 out]
        n207 = property on="窗格" class="Pane"("Origin"=T2 {"Horizontal"=0, "Vertical"=628} ("原点")) -> ()  [unwired: 2 in, 2 out]
        n208 = Index Array(array=w309) -> (element=w310:refnum<vi>)  [unwired: 1 in]
        n209 = property class="VI"(reference=w310) -> (reference out=w306:refnum<vi>, "Exec.State"=w305:T11)  [unwired: 1 in, 1 out]
        n210 = case shown="\"Bad\", 默认" w305 {
          tunnel: [w312 w314] -> w308
          tunnel: w306 -> [w312 w313]
          frame "Bad", Default {
          }
          frame "Idle" {
            n211 = invoke class="VI" method="Run VI"(reference=w313, "Wait until done"=FALSE ("结束前等待"), "Auto Dispose Ref"=FALSE ("自动销毁引用")) -> (reference out=w314:refnum<vi>)  [unwired: 2 in, 4 out]
          }
        }
        n212 = invoke on="参数查询子面板" class="SubPnl" method="Remove VI"() -> (error out=w307:errorcluster)  [unwired: 3 in, 2 out]
        n213 = invoke on="参数查询子面板" class="SubPnl" method="Insert VI"(error in=w307, "VI Ref"=w308) -> ()  [unwired: 2 in, 4 out]
      }
      event "返回": Value Change {
        n214 = event-data() -> ()  [unwired: 1 in, 6 out]
        n215 = property on="窗格" class="Pane"("Origin"=T2 {"Horizontal"=0, "Vertical"=0} ("原点")) -> ()  [unwired: 2 in, 2 out]
        n216 = disable-structure shown="禁用" {
          disable-tunnel: w317 -> [w319 _]
          frame Disabled {
            n217 = for {
              tunnel: w319 -> [w322] mode=indexing
              n218 = property class="VI"(reference=w322) -> (reference out=w320:refnum<vi>, "Exec.State"=w321:T11)  [unwired: 1 in, 1 out]
              n219 = case shown="\"Run top level\"" w321 {
                tunnel: w320 -> [_ _ w323 w324]
                frame "Bad", Default {
                }
                frame "Idle" {
                }
                frame "Run top level" {
                  n220 = invoke class="VI" method="Abort VI"(reference=w323) -> ()  [unwired: 2 in, 3 out]
                }
                frame "Running" {
                  n221 = invoke class="VI" method="Abort VI"(reference=w324) -> ()  [unwired: 2 in, 3 out]
                }
              }
            }
          }
          frame Enabled {
          }
        }
      }
      event "pH参数查询": Value Change {
        n222 = event-data() -> ()  [unwired: 1 in, 6 out]
        n223 = Index Array(array=w329) -> (element=w330:refnum<vi>)  [unwired: 1 in]
        n224 = property class="VI"(reference=w330) -> (reference out=w326:refnum<vi>, "Exec.State"=w325:T11)  [unwired: 1 in, 1 out]
        n225 = case shown="\"Bad\", 默认" w325 {
          tunnel: [w331 w333] -> w328
          tunnel: w326 -> [w331 w332]
          frame "Bad", Default {
          }
          frame "Idle" {
            n226 = invoke class="VI" method="Run VI"(reference=w332, "Wait until done"=FALSE ("结束前等待"), "Auto Dispose Ref"=FALSE ("自动销毁引用")) -> (reference out=w333:refnum<vi>)  [unwired: 2 in, 4 out]
          }
        }
        n227 = invoke on="参数查询子面板" class="SubPnl" method="Remove VI"() -> (error out=w327:errorcluster)  [unwired: 3 in, 2 out]
        n228 = invoke on="参数查询子面板" class="SubPnl" method="Insert VI"(error in=w327, "VI Ref"=w328) -> ()  [unwired: 2 in, 4 out]
      }
      event "电导率参数查询": Value Change {
        n229 = event-data() -> ()  [unwired: 1 in, 6 out]
        n230 = Index Array(array=w341, index=1 ("索引")) -> (element=w342:refnum<vi>)
        n231 = property class="VI"(reference=w342) -> (reference out=w337:refnum<vi>, "Exec.State"=w336:T11)  [unwired: 1 in, 1 out]
        n232 = case shown="\"Bad\", 默认" w336 {
          tunnel: w337 -> [w343 w347]
          tunnel: [w343 w344] -> w339
          frame "Bad", Default {
          }
          frame "Idle" {
            n233 = invoke class="VI" method="Run VI"(reference=w347, "Wait until done"=FALSE ("结束前等待"), "Auto Dispose Ref"=FALSE ("自动销毁引用")) -> (reference out=w344:refnum<vi>)  [unwired: 2 in, 4 out]
          }
        }
        n234 = invoke on="参数查询子面板" class="SubPnl" method="Remove VI"() -> (error out=w338:errorcluster)  [unwired: 3 in, 2 out]
        n235 = invoke on="参数查询子面板" class="SubPnl" method="Insert VI"(error in=w338, "VI Ref"=w339) -> ()  [unwired: 2 in, 4 out]
      }
      event "溶解氧参数查询": Value Change {
        n236 = event-data() -> ()  [unwired: 1 in, 6 out]
        n237 = Index Array(array=w353, index=2 ("索引")) -> (element=w354:refnum<vi>)
        n238 = property class="VI"(reference=w354) -> (reference out=w349:refnum<vi>, "Exec.State"=w348:T11)  [unwired: 1 in, 1 out]
        n239 = case shown="\"Bad\", 默认" w348 {
          tunnel: [w355 w357] -> w351
          tunnel: w349 -> [w355 w356]
          frame "Bad", Default {
          }
          frame "Idle" {
            n240 = invoke class="VI" method="Run VI"(reference=w356, "Wait until done"=FALSE ("结束前等待"), "Auto Dispose Ref"=FALSE ("自动销毁引用")) -> (reference out=w357:refnum<vi>)  [unwired: 2 in, 4 out]
          }
        }
        n241 = invoke on="参数查询子面板" class="SubPnl" method="Remove VI"() -> (error out=w350:errorcluster)  [unwired: 3 in, 2 out]
        n242 = invoke on="参数查询子面板" class="SubPnl" method="Insert VI"(error in=w350, "VI Ref"=w351) -> ()  [unwired: 2 in, 4 out]
      }
      event "浊度参数查询": Value Change {
        n243 = event-data() -> ()  [unwired: 1 in, 6 out]
        n244 = Index Array(array=w365, index=3 ("索引")) -> (element=w366:refnum<vi>)
        n245 = property class="VI"(reference=w366) -> (reference out=w361:refnum<vi>, "Exec.State"=w360:T11)  [unwired: 1 in, 1 out]
        n246 = case shown="\"Bad\", 默认" w360 {
          tunnel: [w367 w369] -> w363
          tunnel: w361 -> [w367 w368]
          frame "Bad", Default {
          }
          frame "Idle" {
            n247 = invoke class="VI" method="Run VI"(reference=w368, "Wait until done"=FALSE ("结束前等待"), "Auto Dispose Ref"=FALSE ("自动销毁引用")) -> (reference out=w369:refnum<vi>)  [unwired: 2 in, 4 out]
          }
        }
        n248 = invoke on="参数查询子面板" class="SubPnl" method="Remove VI"() -> (error out=w362:errorcluster)  [unwired: 3 in, 2 out]
        n249 = invoke on="参数查询子面板" class="SubPnl" method="Insert VI"(error in=w362, "VI Ref"=w363) -> ()  [unwired: 2 in, 4 out]
      }
      event "水温校准": Value Change {
        n250 = event-data() -> ()  [unwired: 1 in, 6 out]
        n251 = Index Array(array=w377, index=4 ("索引")) -> (element=w378:refnum<vi>)
        n252 = property class="VI"(reference=w378) -> (reference out=w373:refnum<vi>, "Exec.State"=w372:T11)  [unwired: 1 in, 1 out]
        n253 = case shown="\"Bad\", 默认" w372 {
          tunnel: [w379 w381] -> w375
          tunnel: w373 -> [w379 w380]
          frame "Bad", Default {
          }
          frame "Idle" {
            n254 = invoke class="VI" method="Run VI"(reference=w380, "Wait until done"=FALSE ("结束前等待"), "Auto Dispose Ref"=FALSE ("自动销毁引用")) -> (reference out=w381:refnum<vi>)  [unwired: 2 in, 4 out]
          }
        }
        n255 = invoke on="探头校准子面板" class="SubPnl" method="Remove VI"() -> (error out=w374:errorcluster)  [unwired: 3 in, 2 out]
        n256 = invoke on="探头校准子面板" class="SubPnl" method="Insert VI"(error in=w374, "VI Ref"=w375) -> ()  [unwired: 2 in, 4 out]
      }
      event "pH校准": Value Change {
        n257 = event-data() -> ()  [unwired: 1 in, 6 out]
        n258 = Index Array(array=w389, index=5 ("索引")) -> (element=w390:refnum<vi>)
        n259 = property class="VI"(reference=w390) -> (reference out=w385:refnum<vi>, "Exec.State"=w384:T11)  [unwired: 1 in, 1 out]
        n260 = case shown="\"Bad\", 默认" w384 {
          tunnel: w385 -> [w391 w395]
          tunnel: [w391 w392] -> w387
          frame "Bad", Default {
          }
          frame "Idle" {
            n261 = invoke class="VI" method="Run VI"(reference=w395, "Wait until done"=FALSE ("结束前等待"), "Auto Dispose Ref"=FALSE ("自动销毁引用")) -> (reference out=w392:refnum<vi>)  [unwired: 2 in, 4 out]
          }
        }
        n262 = invoke on="探头校准子面板" class="SubPnl" method="Remove VI"() -> (error out=w386:errorcluster)  [unwired: 3 in, 2 out]
        n263 = invoke on="探头校准子面板" class="SubPnl" method="Insert VI"(error in=w386, "VI Ref"=w387) -> ()  [unwired: 2 in, 4 out]
      }
      event "电导率校准": Value Change {
        n264 = event-data() -> ()  [unwired: 1 in, 6 out]
        n265 = Index Array(array=w401, index=6 ("索引")) -> (element=w402:refnum<vi>)
        n266 = property class="VI"(reference=w402) -> (reference out=w397:refnum<vi>, "Exec.State"=w396:T11)  [unwired: 1 in, 1 out]
        n267 = case shown="\"Bad\", 默认" w396 {
          tunnel: [w403 w405] -> w399
          tunnel: w397 -> [w403 w404]
          frame "Bad", Default {
          }
          frame "Idle" {
            n268 = invoke class="VI" method="Run VI"(reference=w404, "Wait until done"=FALSE ("结束前等待"), "Auto Dispose Ref"=FALSE ("自动销毁引用")) -> (reference out=w405:refnum<vi>)  [unwired: 2 in, 4 out]
          }
        }
        n269 = invoke on="探头校准子面板" class="SubPnl" method="Remove VI"() -> (error out=w398:errorcluster)  [unwired: 3 in, 2 out]
        n270 = invoke on="探头校准子面板" class="SubPnl" method="Insert VI"(error in=w398, "VI Ref"=w399) -> ()  [unwired: 2 in, 4 out]
      }
      event "溶解氧校准": Value Change {
        n271 = event-data() -> ()  [unwired: 1 in, 6 out]
        n272 = Index Array(array=w413, index=7 ("索引")) -> (element=w414:refnum<vi>)
        n273 = property class="VI"(reference=w414) -> (reference out=w409:refnum<vi>, "Exec.State"=w408:T11)  [unwired: 1 in, 1 out]
        n274 = case shown="\"Bad\", 默认" w408 {
          tunnel: [w415 w417] -> w411
          tunnel: w409 -> [w415 w416]
          frame "Bad", Default {
          }
          frame "Idle" {
            n275 = invoke class="VI" method="Run VI"(reference=w416, "Wait until done"=FALSE ("结束前等待"), "Auto Dispose Ref"=FALSE ("自动销毁引用")) -> (reference out=w417:refnum<vi>)  [unwired: 2 in, 4 out]
          }
        }
        n276 = invoke on="探头校准子面板" class="SubPnl" method="Remove VI"() -> (error out=w410:errorcluster)  [unwired: 3 in, 2 out]
        n277 = invoke on="探头校准子面板" class="SubPnl" method="Insert VI"(error in=w410, "VI Ref"=w411) -> ()  [unwired: 2 in, 4 out]
      }
      event "浊度校准": Value Change {
        n278 = event-data() -> ()  [unwired: 1 in, 6 out]
        n279 = Index Array(array=w425, index=8 ("索引")) -> (element=w426:refnum<vi>)
        n280 = property class="VI"(reference=w426) -> (reference out=w421:refnum<vi>, "Exec.State"=w420:T11)  [unwired: 1 in, 1 out]
        n281 = case shown="\"Bad\", 默认" w420 {
          tunnel: [w427 w429] -> w423
          tunnel: w421 -> [w427 w428]
          frame "Bad", Default {
          }
          frame "Idle" {
            n282 = invoke class="VI" method="Run VI"(reference=w428, "Wait until done"=FALSE ("结束前等待"), "Auto Dispose Ref"=FALSE ("自动销毁引用")) -> (reference out=w429:refnum<vi>)  [unwired: 2 in, 4 out]
          }
        }
        n283 = invoke on="探头校准子面板" class="SubPnl" method="Remove VI"() -> (error out=w422:errorcluster)  [unwired: 3 in, 2 out]
        n284 = invoke on="探头校准子面板" class="SubPnl" method="Insert VI"(error in=w422, "VI Ref"=w423) -> ()  [unwired: 2 in, 4 out]
      }
      event "叶绿素a校准": Value Change {
        n285 = event-data() -> ()  [unwired: 1 in, 6 out]
        n286 = Index Array(array=w437, index=9 ("索引")) -> (element=w438:refnum<vi>)
        n287 = property class="VI"(reference=w438) -> (reference out=w433:refnum<vi>, "Exec.State"=w432:T11)  [unwired: 1 in, 1 out]
        n288 = case shown="\"Bad\", 默认" w432 {
          tunnel: [w439 w441] -> w435
          tunnel: w433 -> [w439 w440]
          frame "Bad", Default {
          }
          frame "Idle" {
            n289 = invoke class="VI" method="Run VI"(reference=w440, "Wait until done"=FALSE ("结束前等待"), "Auto Dispose Ref"=FALSE ("自动销毁引用")) -> (reference out=w441:refnum<vi>)  [unwired: 2 in, 4 out]
          }
        }
        n290 = invoke on="探头校准子面板" class="SubPnl" method="Remove VI"() -> (error out=w434:errorcluster)  [unwired: 3 in, 2 out]
        n291 = invoke on="探头校准子面板" class="SubPnl" method="Insert VI"(error in=w434, "VI Ref"=w435) -> ()  [unwired: 2 in, 4 out]
      }
    }
  }
